vi "NI_FPGA_PPG.ProcEvents.vi"(0 "i ref in":refnum<vi>, 5 "error in (no error)":errorcluster) -> (14 "i ref out":refnum<vi>, 19 "error out":errorcluster)   [LabVIEW 2014, in "NI_FPGA_PPG.lvlib"]
doc: "This method is used to define the events the object will listen to. Add your own events here."
uses:
  NI_FPGA_PPG.lvlib
  CSCore/BaseProcess/BaseProcess.event definition.ctl
  CSCore/CAEObj/CAEObj.event definition.ctl
  CSCore/BaseProcess/BaseProcess.descriptor string definition.ctl
  CSCore/BaseProcess/BaseProcess.lvlib
  CSCore/CAEObj/CAEObj.lvlib
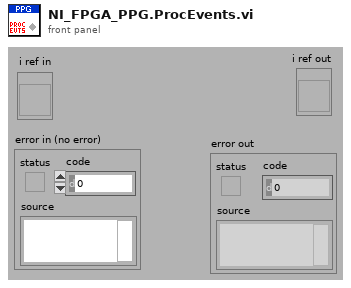
[diagram p1: front panel]
types:
  T1 = typedef "BaseProcess.lvlib/BaseProcess.event definition.ctl" = cluster{"CAEEvtDef":T2, "Data Descriptor":T3}
  T2 = typedef "CAEObj.lvlib/CAEObj.event definition.ctl" = cluster{"URL":string, "enable":bool, "ignoreResID":bool}
  T3 = typedef "BaseProcess.lvlib/BaseProcess.descriptor string definition.ctl" = string
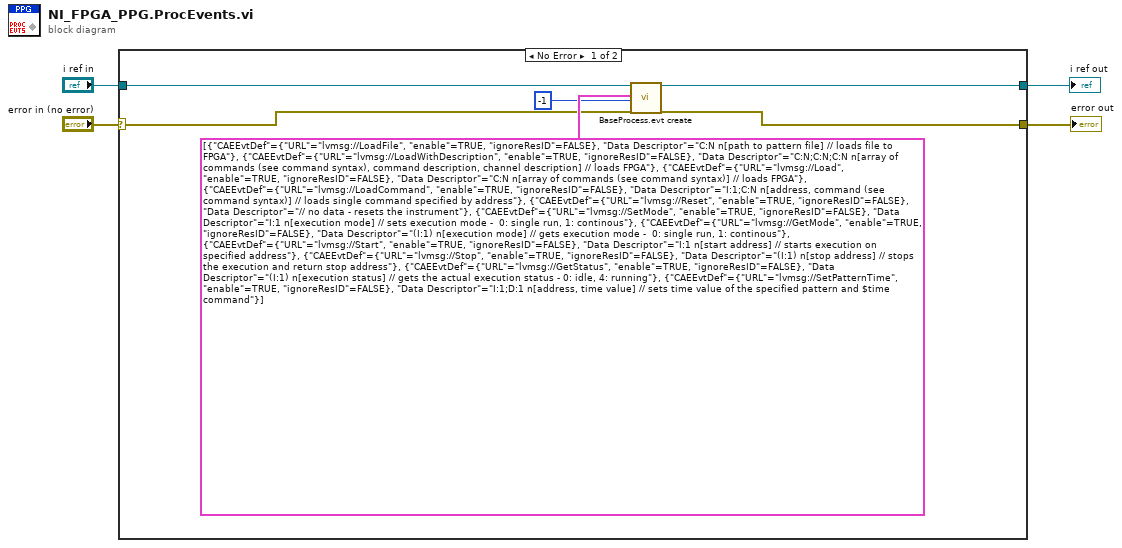
[diagram p0: block diagram]
diagram:
  n1 = case shown="No Error" "error in (no error)" {
    selector: "error in (no error)" -> [w6 w11]
    tunnel: "i ref in" -> [w10 w12]
    tunnel: [w9 w12] -> w3
    tunnel: [w8 w11] -> w2
    frame No Error {
      n2 = call "BaseProcess.evt create.vi"("i ref in"=w10, "newEvents"=T1[] [{"CAEEvtDef"={"URL"="lvmsg://LoadFile", "enable"=TRUE, "ignoreResID"=FALSE}, "Data Descriptor"="C:N n[path to pattern file] // loads file to FPGA"}, {"CAEEvtDef"={"URL"="lvmsg://LoadWithDescription", "enable"=TRUE, "ignoreResID"=FALSE}, "Data Descriptor"="C:N;C:N;C:N n[array of commands (see command syntax), command description, channel description] // loads FPGA"}, {"CAEEvtDef"={"URL"="lvmsg://Load", "enable"=TRUE, "ignoreResID"=FALSE}, "Data Descriptor"="C:N n[array of commands (see command syntax)] // loads FPGA"}, {"CAEEvtDef"={"URL"="lvmsg://LoadCommand", "enable"=TRUE, "ignoreResID"=FALSE}, "Data Descriptor"="I:1;C:N n[address, command (see command syntax)] // loads single command specified by address"}, {"CAEEvtDef"={"URL"="lvmsg://Reset", "enable"=TRUE, "ignoreResID"=FALSE}, "Data Descriptor"="// no data - resets the instrument"}, {"CAEEvtDef"={"URL"="lvmsg://SetMode", "enable"=TRUE, "ignoreResID"=FALSE}, "Data Descriptor"="I:1 n[execution mode] // sets execution mode -  0: single run, 1: continous"}, {"CAEEvtDef"={"URL"="lvmsg://GetMode", "enable"=TRUE, "ignoreResID"=FALSE}, "Data Descriptor"="(I:1) n[execution mode] // gets execution mode -  0: single run, 1: continous"}, {"CAEEvtDef"={"URL"="lvmsg://Start", "enable"=TRUE, "ignoreResID"=FALSE}, "Data Descriptor"="I:1 n[start address] // starts execution on specified address"}, {"CAEEvtDef"={"URL"="lvmsg://Stop", "enable"=TRUE, "ignoreResID"=FALSE}, "Data Descriptor"="(I:1) n[stop address] // stops the execution and return stop address"}, {"CAEEvtDef"={"URL"="lvmsg://GetStatus", "enable"=TRUE, "ignoreResID"=FALSE}, "Data Descriptor"="(I:1) n[execution status] // gets the actual execution status - 0: idle, 4: running"}, {"CAEEvtDef"={"URL"="lvmsg://SetPatternTime", "enable"=TRUE, "ignoreResID"=FALSE}, "Data Descriptor"="I:1;D:1 n[address, time value] // sets time value of the specified pattern and $time command"}] ("new events"), "ms timeout (10000)"=-1, "error in (no error)"=w6) -> ("i ref out"=w9:refnum<vi>, "error out"=w8:errorcluster)  [unwired: 12 in, 2 out]
    }
    frame Error {
    }
  }
  "i ref out" <- w3
  "error out" <- w2
